vi "get_block_size.vi"(8 "error in (no error)":errorcluster, 11 "DL090202ScanHead in":refnum<class "ScanHeadDL090202.lvclass">) -> (0 "error out":errorcluster, 2 "block size":i32, 3 "DL090202ScanHead out":refnum<class "ScanHeadDL090202.lvclass">)   [LabVIEW 2010]
uses:
  ScanHeadDL090202.lvclass
  Trajectory/TrajectoryDL091126GenericVoxel/TrajectoryDL091126GenericVoxel/TrajectoryDL091126GenericVoxel.lvclass
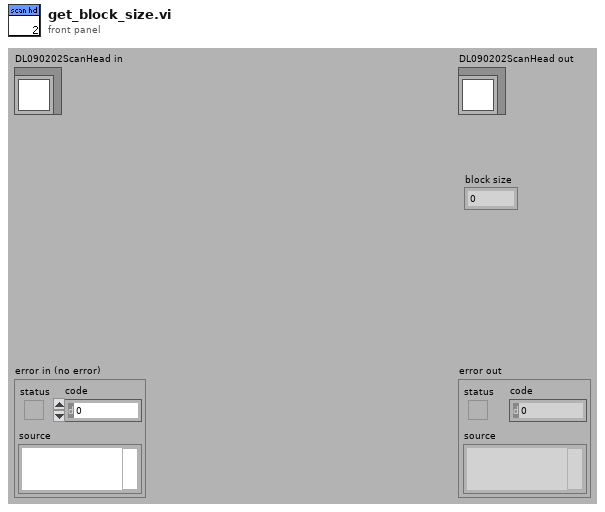
[diagram p1: front panel]
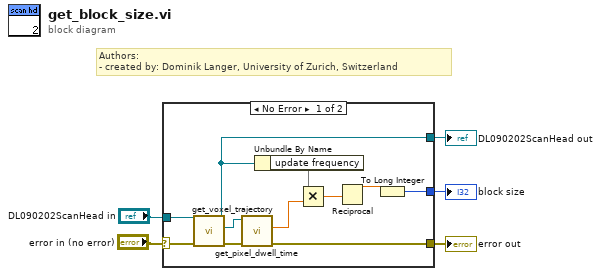
[diagram p0: block diagram]
diagram:
  # "Authors: \n- created by: Dominik Langer, University of Zurich, Switzerland"
  n1 = case shown="No Error" "error in (no error)" {
    selector: "error in (no error)" -> [w12 w18]
    tunnel: [w11 w18] -> w4
    tunnel: [w9 w17] -> w2
    tunnel: "DL090202ScanHead in" -> [w10 w17]
    tunnel: [w6 _] -> w1
    frame No Error {
      n2 = call-dynamic "get_voxel_trajectory.vi"("error in (no error)"=w12, "ScanHeadDL090202 in"=w10) -> ("error out"=w13:errorcluster, "trajectory"=w16:refnum<class "TrajectoryDL091126GenericVoxel.lvclass">, "ScanHeadDL090202 out"=w9:refnum<class "ScanHeadDL090202.lvclass">)  [unwired: 7 in]
      n3 = call-dynamic "get_pixel_dwell_time.vi"("error in (no error)"=w13, "GenericTrajectory.lvclass in"=w16) -> ("error out"=w11:errorcluster, "pixel dwell time"=w15:dbl[unit])  [unwired: 7 in, 1 out]
      n4 = Unbundle By Name(w9) -> ("update frequency"=w14)
      n5 = Multiply(x=w14, y=w15) -> (x*y=w8:dbl[unit])
      n6 = Reciprocal(x=w8) -> (1/x=w7:dbl[unit])
      n7 = To Long Integer(number=w7) -> (32bit integer=w6:i32)
    }
    frame Error {
    }
  }
  "error out" <- w4
  "DL090202ScanHead out" <- w2
  "block size" <- w1
